vi "PCO_whisker_puff_pupil_FLIR_trig_2024_JMR.vi"() -> ()   [LabVIEW 2020]
uses:
  C:/Users/jqr5792/AppData/Roaming/PCO Digital Camera Toolbox/pco.labview/pco.camera/Controls/binning.ctl
  <vilib>/vision/driver/IMAQdx.llb/IMAQdx Camera Control Mode.ctl
  <vilib>/userDefined/High Color/IMAQdx.ctl
  <vilib>/vision/driver/IMAQdx.llb/IMAQdx Acquisition Mode.ctl
  C:/Users/jqr5792/AppData/Roaming/PCO Digital Camera Toolbox/pco.labview/pco.camera/Camera.lvclass
  <vilib>/vision/driver/IMAQdx.llb/IMAQdx Buffer Number Mode.ctl
  <vilib>/DAQmx/write.llb/DAQmx Write (Digital Bool 1Line 1Point).vi
  <vilib>/DAQmx/read.llb/DAQmx Read (Analog 1D Wfm NChan NSamp).vi
  <vilib>/DAQmx/write.llb/DAQmx Write (Digital 1D Bool NChan 1Samp 1Line).vi
  <vilib>/DAQmx/create/channels.llb/DAQmx Create Channel (AI-Voltage-Basic).vi
  <vilib>/DAQmx/configure/timing.llb/DAQmx Timing (Sample Clock).vi
  <vilib>/DAQmx/configure/trigger.llb/DAQmx Start Trigger (Digital Edge).vi
  <vilib>/DAQmx/create/channels.llb/DAQmx Create Channel (DO-Digital Output).vi
  <vilib>/DAQmx/create/channels.llb/DAQmx Create Channel (CO-Pulse Generation-Frequency).vi
  <vilib>/DAQmx/configure/timing.llb/DAQmx Timing (Implicit).vi
  <vilib>/DAQmx/miscellaneous.llb/DAQmx Fill In Error Info.vi
  <vilib>/vision/driver/NI_Vision_Acquisition_Software.lvlib
panel:
  out "n total images":i32
  out "PCO Frame Rate":dbl
  out "Time Elapsed (s)":u32
  out "Recorded Images":u32=7194
  out "PCO Recording":bool=TRUE
  in  "ROI":cluster{"x0":u64, "y0":u64, "x1":u64, "y1":u64}={"x0"=100, "y0"=175, "x1"=500, "y1"=425}
  in  "Binning":T1={"vert"=4, "horz"=4}
  in  "TriggerMode":T2(ring)=enum."external exposure start"
  in  "Exposure [s]":dbl=0.008 min=0.0005 max=2.0 step=0.001
  out "Image":T3(plugin-control)
  out "Last Whisk\nBuffer":u32=488
  out "Actual WhiskCam\nFrame Rate":dbl(knob)=148.05583250249254 scale=0.0..300.0
  out "Pupil":T3(plugin-control)
  out "Solenoids":bool[](array[boolean])
  in  "Stim \nOffset (s)":dbl=15.0
  in  "Stim \nDuration (s)":dbl=0.1 step=0.1
  in  "Inter-Stim\nInterval (s)":dbl=30.0
  in  "Right Pad 2":dbl=1.0
  in  "Left Pad 2":dbl=5.0
  in  "Control 2":dbl=2.0
  in  "Left Pad":tag="Dev1/port0/line1"
  in  "Right Pad":tag="Dev1/port0/line3"
  in  "Control":tag="Dev1/port0/line2"
  out "Analog Data":bool
  out "Analog acquisition length":i32
  in  "Channel Labels":string[](array[string])=["BallVelocity", "LeftPad", "Control", "RightPad", "Broadband", "LFP", "MUA"]
  in  "physical channels":tag="Dev1/ai0:6"
  in  "Analog Acquisition Setup":cluster{"Analog Sampling Rate":u16}={"Analog Sampling Rate"=5000} {"Analog Sampling Rate" format="%0.0f"}
  in  "Camera Acquisition Setup":cluster{"CBVCam Rate":u16, "WebCam Rate":u16}={"CBVCam Rate"=60, "WebCam Rate"=30}
  out "Notes Size":i32=7
  out "Notes Reversed":string[](array[string])=["Experimenter", "Animal ID", "Imaged Hemisphere", "Solenoid Pressure", "Isoflurane time", "Session ID", "Amplifier Gain"]
  out "Notes Array":string[](array[string])=["Amplifier Gain", "Session ID", "Isoflurane time", "Solenoid Pressure", "Imaged Hemisphere", "Animal ID", "Experimenter"]
  in  "Session Notes:":T4={"Experimenter"="Joe Ricotta", "Animal ID"="T31", "Imaged Hemisphere"="RH", "Solenoid Pressure"="10", "Infusion Compound"="na", "Infusion volume nL"="na", "Infusion rate nlpS"="na", "Block"="1000", "Molar conc um"="na"}
  in  "Target Path":path=path "D:/Joe/sample/PCO_setup" caption="Final saved file location"
  out "Current file name":string="170828_12_37_58"
  out "Actual WebCam Frame Rate":dbl(knob) scale=0.0..30.0
  out "WebCam":T3(plugin-control)
  out "CBV Camera":bool=TRUE
  out "Trial Time Elapsed (Min)":cluster{dbl, dbl}(slide)={0.5, 0.05364406000000001} scale=0.0..20.0
  in  "Recording Time (min)":dbl(knob)=5.0 min=0.5 max=25.0 step=0.5 scale=0.0..25.0 scale format="%#_2g"
  in  "Temp Path":path=path "C:/LabView Direct Files" caption="Temporary path for\nstreamed data"
  in  "Stop":bool
  # "File Settings:"
  # "Binning: 4,4"
  # "roi: 50, 200, 600, 400"
  # "Left Pad"
  # "Control"
  # "Right"
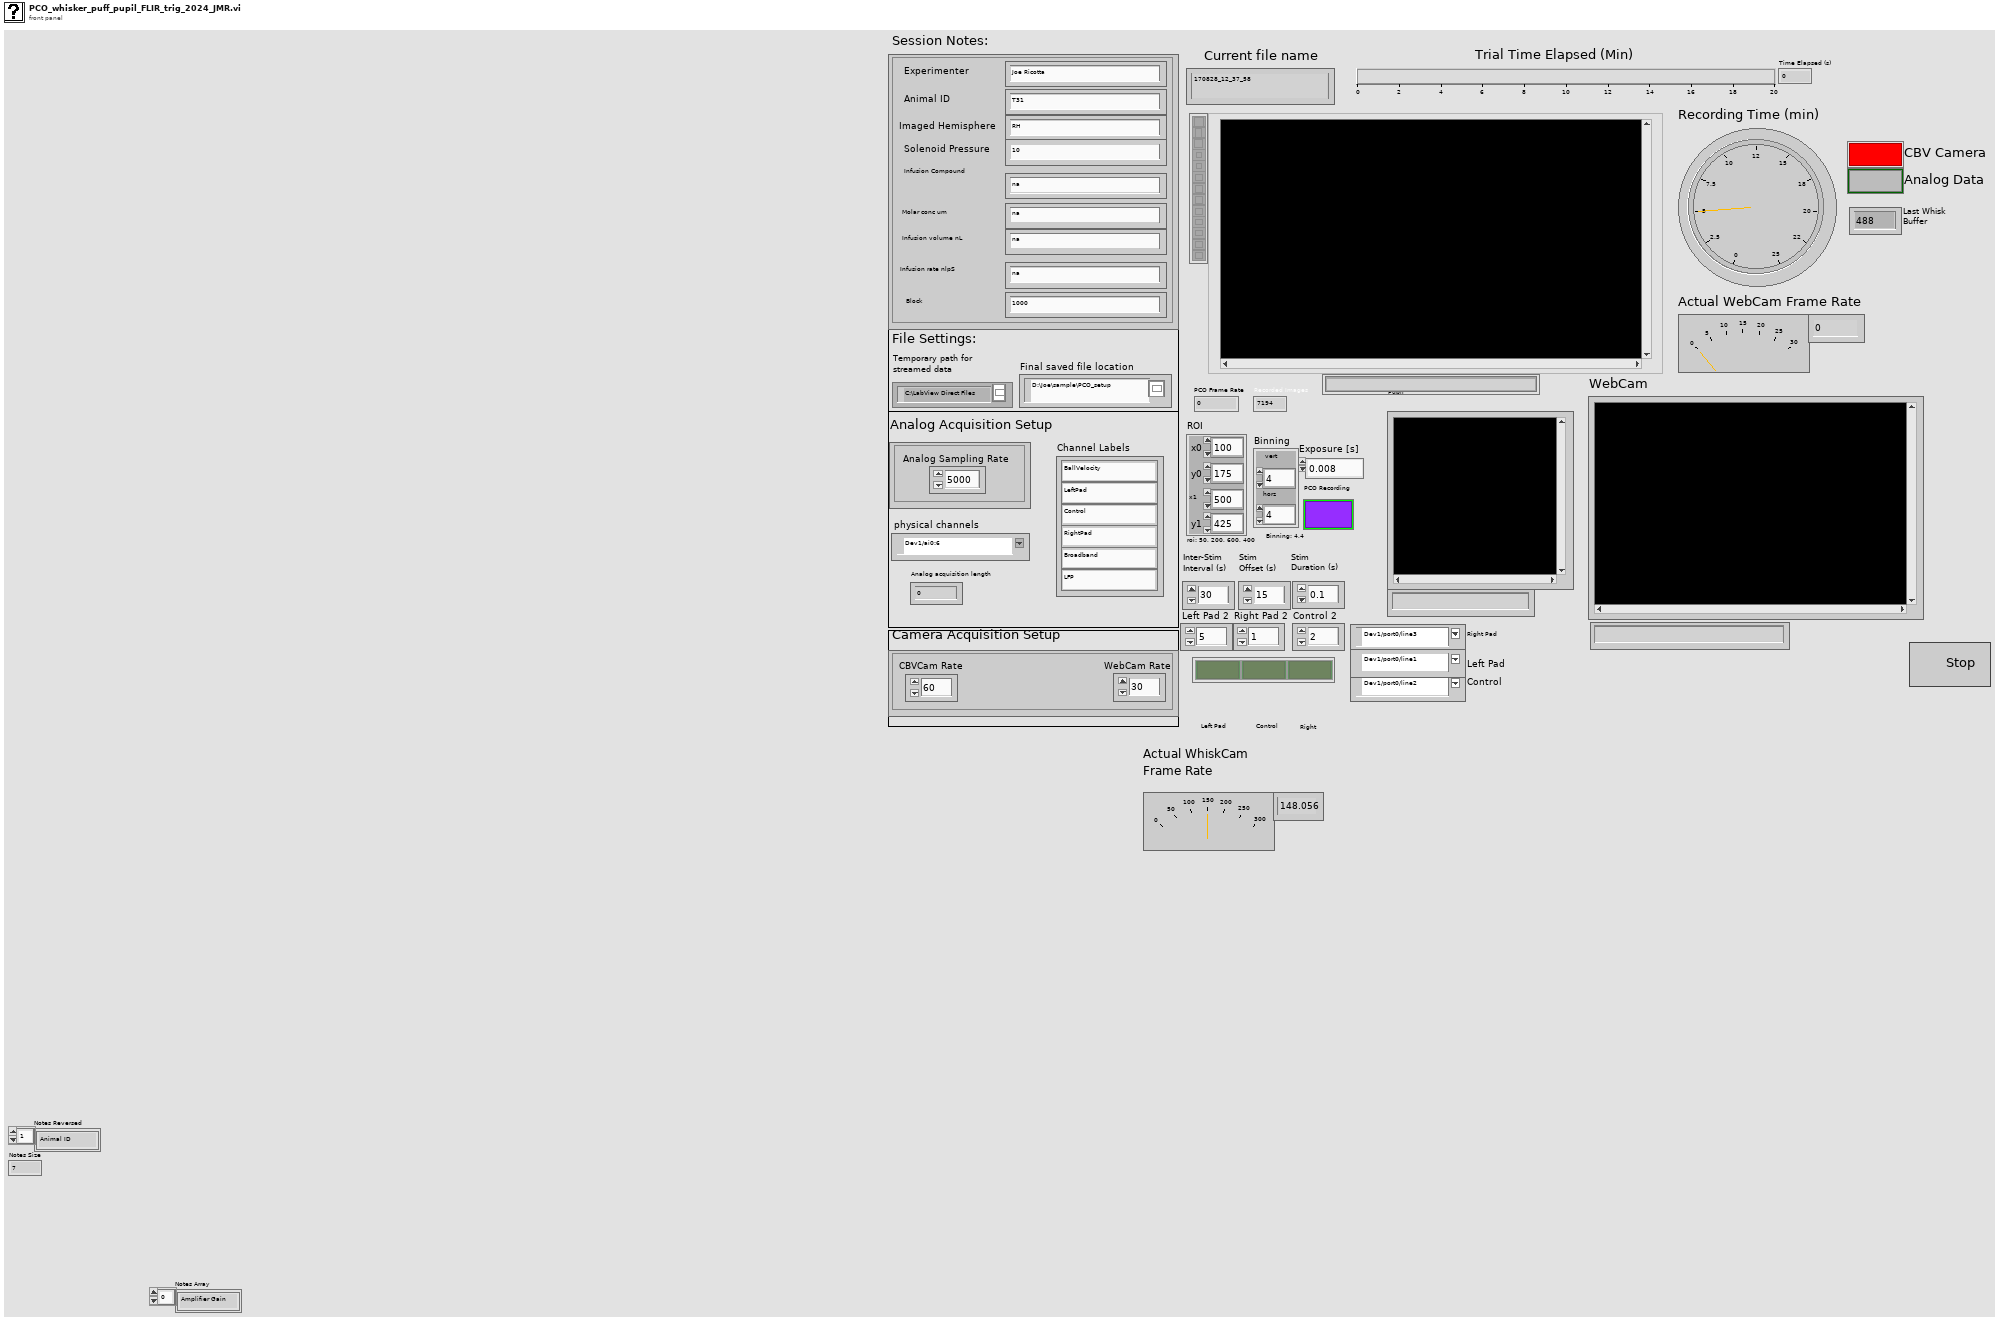
[diagram p1: front panel]
types:
  T1 = typedef "Camera.lvclass/binning.ctl" = cluster{"vert":u16, "horz":u16}
  T2 = enum16{"auto sequence", "software trigger", "external exposure start", "external exposure control"}
  T3 = typedef "IMAQ Image.ctl" = refnum<image>
  T4 = cluster{"Experimenter":string, "Animal ID":string, "Imaged Hemisphere":string, "Solenoid Pressure":string, "Infusion Compound":string, "Infusion volume nL":string, "Infusion rate nlpS":string, "Block":string, "Molar conc um":string}
  T5 = typedef "IMAQdx.ctl" = refnum<k21>
  T6 = typedef "Image Type" = u32
  T7 = enum16{"open", "replace", "create", "open or create", "replace or create", "replace or create with confirmation"}
  T8 = typedef "NI_Vision_Acquisition_Software.lvlib/IMAQdx Acquisition Mode.ctl" = enum32{"One Shot", "Continuous"}
  T9 = typedef "NI_Vision_Acquisition_Software.lvlib/IMAQdx Camera Control Mode.ctl" = enum32{"Controller", "Listener"}
  T10 = enum16{"open", "open or create", "create or replace", "create", "open (read-only)"}
  T11 = cluster{"exposure_time_s":dbl, "delay_time_s":dbl, "roi":cluster{"x0":u64, "y0":u64, "x1":u64, "y1":u64}, "timestamp_mode":u16, "pixelrate":u32, "trigger_mode":u16, "acquire_mode":u16, "metadata_mode":u16, "noisefilter_mode":u16, "binning":T1}
  T12 = typedef "IMAQ AVI2 Refnum.ctl" = refnum<k20>
  T13 = enum16{"sequence", "sequence non blocking", "ring buffer", "fifo", "sequence_dpcore", "sequence_non_blocking_dpcore", "ring_buffer_dpcore", "fifo_dpcore", "tif", "multitif", "pcoraw", "b16", "dicom", "multidicom"}
  T14 = enum16{"Undefined", "Mono8", "Mono16", "BGRA8", "RGBA8", "BGRA16", "RGBA16", "CompressedMono8"}
  T15 = enum16{"big-endian, network order", "native, host order", "little-endian"}
  T16 = typedef "NI_Vision_Acquisition_Software.lvlib/IMAQdx Buffer Number Mode.ctl" = enum32{"Next", "Last", "Buffer Number", "Every", "Last New"}
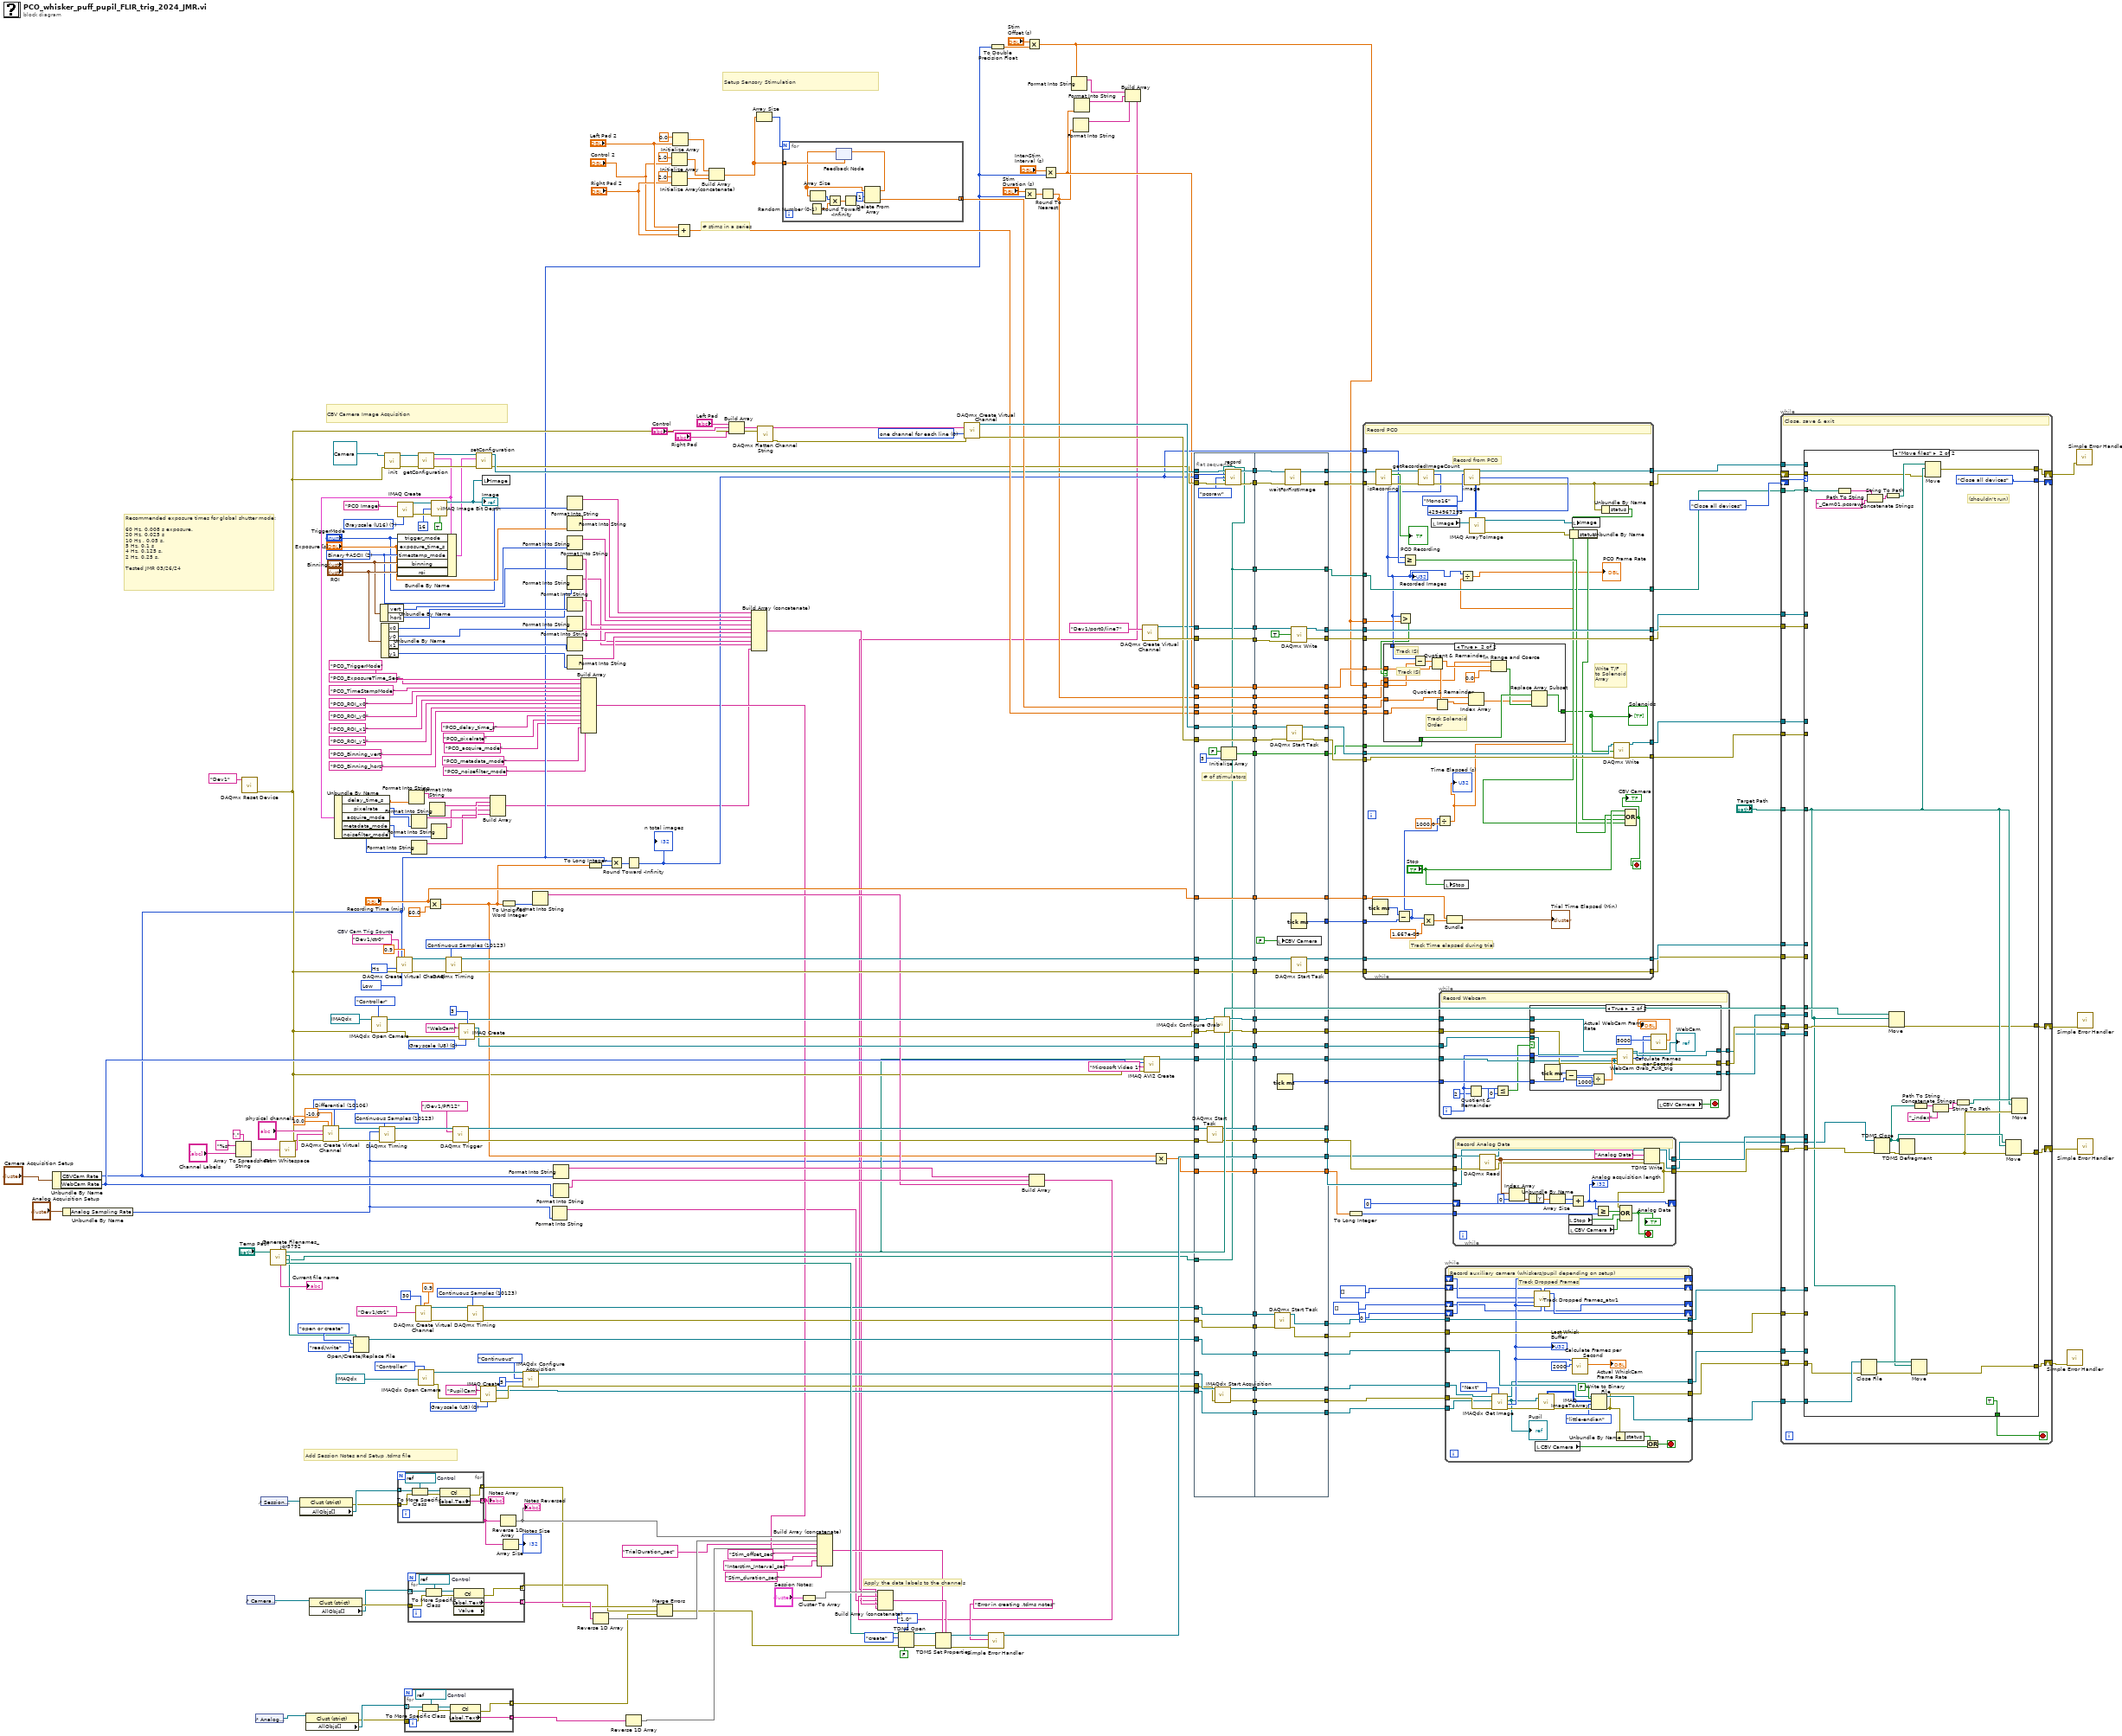
[diagram p0: block diagram]
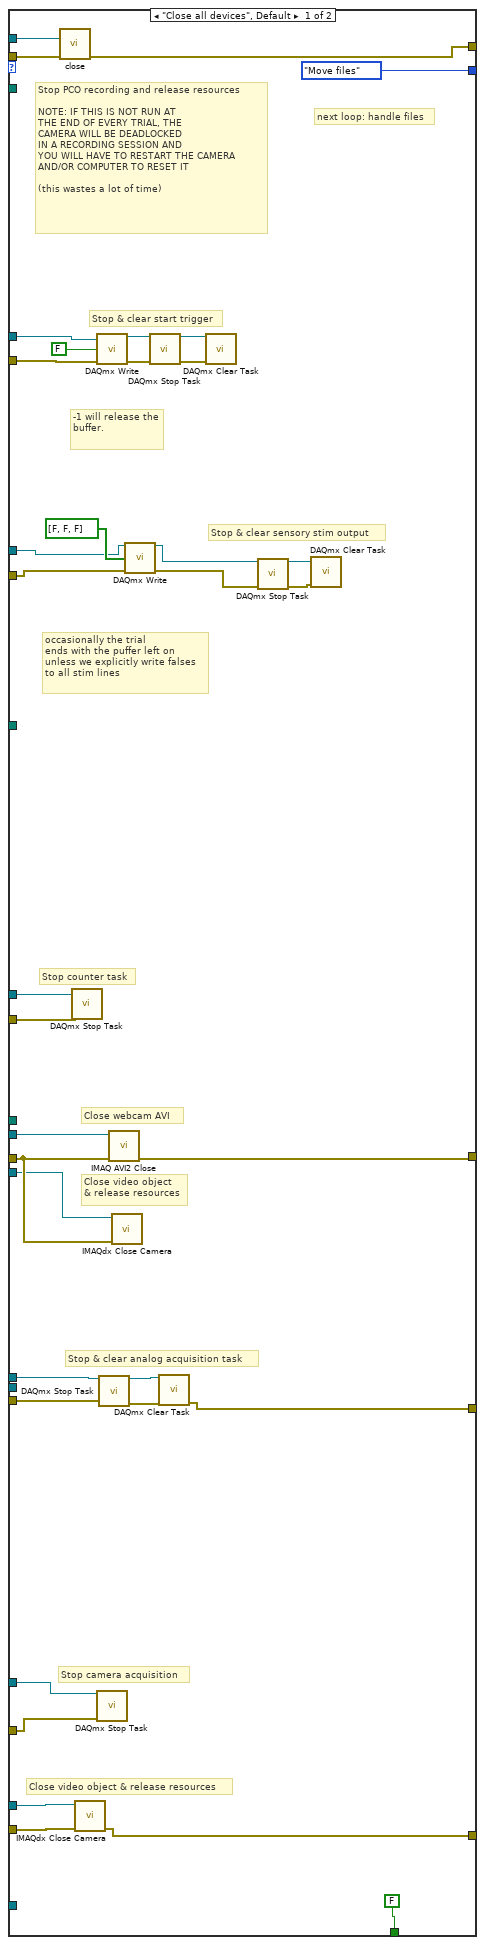
[diagram p2: hidden frame]
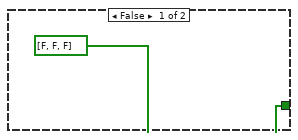
[diagram p4: hidden frame]
diagram:
  w84 = u16 2 items=["OFF", "Binary", "Binary+ASCII", "ASCII"] ("wTimeStampMode")
  w118 = T6 7 items=["Grayscale (U8)", "Grayscale (I16)", "Grayscale (SGL)", "Complex (CSG)", "RGB (U32)", "HSL (U32)", "RGB (U64)", "Grayscale (U16)"] ("Image Type")
  w148 = 10123 items=["Finite Samples"=10178, "Continuous Samples"=10123, "Hardware Timed Single Point"=12522] ("sample mode")
  w153 = T6 0 items=["Grayscale (U8)", "Grayscale (I16)", "Grayscale (SGL)", "Complex (CSG)", "RGB (U32)", "HSL (U32)", "RGB (U64)", "Grayscale (U16)"] ("Image Type")
  w203 = 0 items=["one channel for each line", "one channel for all lines"] ("line grouping")
  w206 = tag "Dev1/ctr0"  # CBV Cam Trig Source
  w280 = 10123 items=["Finite Samples"=10178, "Continuous Samples"=10123, "Hardware Timed Single Point"=12522] ("sample mode")
  w283 = 10106 items=["default"=-1, "RSE"=10083, "NRSE"=10078, "Differential"=10106, "Pseudodifferential"=12529] ("input terminal configuration")
  w303 = T6 0 items=["Grayscale (U8)", "Grayscale (I16)", "Grayscale (SGL)", "Complex (CSG)", "RGB (U32)", "HSL (U32)", "RGB (U64)", "Grayscale (U16)"] ("Image Type")
  w309 = 10123 items=["Finite Samples"=10178, "Continuous Samples"=10123, "Hardware Timed Single Point"=12522] ("sample mode")
  w312 = 10373 items=["Hz"=10373] ("units")
  w313 = 10214 items=["High"=10192, "Low"=10214] ("idle state")
  # "Recommended exposure times for global shutter mode:\n\n60 Hz, 0.008 s exposure.\n20 Hz, 0.025 s\n10 Hz , 0.05 s.\n5 Hz, 0.1 s\n4 Hz, 0.125 s.\n2 Hz, 0.25 s.\n\nTested JMR 03/26/24"
  # "Setup Sensory Stimulation"
  # "# stims in a series"
  # "Apply the data labels to the channels"
  # "CBV Camera Image Acquisition"
  # "Add Session Notes and Setup .tdms file"
  n1 = Unbundle By Name "Unbundle By Name"("Camera Acquisition Setup") -> ("CBVCam Rate"=w31:u16, "WebCam Rate"=w124:u16)
  n2 = Unbundle By Name("Analog Acquisition Setup") -> ("Analog Sampling Rate"=w29:u16)
  n3 = Array To Spreadsheet String(delimiter (Tab)=",", array="Channel Labels", 3:"%s" ("format string")) -> (spreadsheet string=w221:string)
  n4 = call <vilib>:"DAQmx Reset Device.vi"("device in"=tag "Dev1") -> ("error out"=w66:errorcluster)  [unwired: 14 in]
  n5 = control-ref of="Camera Acquisition Setup"() -> (w234:refnum<vi>)
  n6 = control-ref of="Analog Acquisition Setup"() -> (w233:refnum<vi>)
  n7 = control-ref of="Session Notes:"() -> (w257:refnum<vi>)
  n8 = call "Generate Filenames_jqr5792.vi"("path"="Temp Path") -> ("TDMS Path"=w251:path, "PCO Path"=w77:path, "Basler Path"=w145:path, "WebCam Path"=w44:path, "Analog file name"=→"Current file name":string)  [unwired: 5 in, 1 out]
  n9 = call <vilib>:"Trim Whitespace.vi"("string"=w221) -> ("trimmed string"=w220:string)  [unwired: 1 in]
  n10 = property class="Clust (strict)"(reference=w257) -> (error out=w260:errorcluster, "AllObjs[]"=w261:refnum<vi>[])  [unwired: 1 in, 1 out]
  n11 = property class="Clust (strict)"(reference=w233) -> (error out=w231:errorcluster, "AllObjs[]"=w232:refnum<vi>[])  [unwired: 1 in, 1 out]
  n12 = property class="Clust (strict)"(reference=w234) -> (error out=w255:errorcluster, "AllObjs[]"=w254:refnum<vi>[])  [unwired: 1 in, 1 out]
  n13 = call-poly <vilib>:"DAQmx Create Virtual Channel.vi"("maximum value"=10.0, "minimum value"=-10.0, "input terminal configuration"=w283, "physical channels"="physical channels", "name to assign"=w220, "error in"=w66) -> ("task out"=w282:refnum<k21>, "error out"=w281:errorcluster)  [unwired: 8 in]
  n14 = Open/Create/Replace File(file path (use dialog)=w145, operation (0:open)=T7."open or create", access (0:read/write)=enum16{"read/write", "read-only", "write-only"}."read/write") -> (refnum out=w129:refnum<file>)  [unwired: 3 in, 2 out]
  n15 = call <vilib>:"IMAQdx Open Camera.vi"("Camera Control Mode"=IMAQdx_Camera_Control_Mode."Controller", "error in"=w66, "Session In"=T5 "cam9") -> ("error out"=w300:errorcluster, "Session Out"=w298:T5)  [unwired: 7 in]
  n16 = call-poly <vilib>:"DAQmx Timing.vi"("task/channels in"=w282, "sample mode"=w280, "rate"=w29, "error in"=w281) -> ("task out"=w279:refnum<k21>, "error out"=w278:errorcluster)  [unwired: 10 in]
  n17 = Unbundle By Name("Binning") -> ("vert"=w85:u16, "horz"=w86:u16)
  n18 = Unbundle By Name("ROI") -> ("x0"=w87:u64, "y0"=w88:u64, "x1"=w89:u64, "y1"=w90:u64)
  n19 = call-dynamic "init.vi"("Camera in"=refnum<class "Camera.lvclass"> refnum ("PCOCamera in"), "error in (no error)"=w66) -> ("Camera out"=w112:refnum<class "Camera.lvclass">, "error out"=w111:errorcluster)  [unwired: 7 in]
  n20 = call-poly <vilib>:"DAQmx Create Virtual Channel.vi"("frequency"=w31, "duty cycle"=0.9, "counter"=w206, "units"=w312, "error in"=w66, "idle state"=w313) -> ("task out"=w311:refnum<k21>, "error out"=w310:errorcluster)  [unwired: 8 in]
  n21 = call "IMAQ Create"("Image Name"="PCO Image", "Image Type"=w118) -> ("New Image"=w117:T3, "error out"=w116:errorcluster)  [unwired: 3 in]
  n22 = for {
    tunnel: [w318] -> w259 mode=indexing
    tunnel: w261 -> [w317] mode=indexing
    tunnel: w260 -> [w316]
    tunnel: [w314] -> w240 mode=indexing
    w319 = refnum<vi> refnum  # Control
    n23 = To More Specific Class(target class=w319, reference=w317, error in=w316) -> (specific class reference=w320:refnum<vi>, error out=w315:errorcluster)
    n24 = property class="Ctl"(reference=w320, error in=w315) -> (error out=w314:errorcluster, "Label.Text"=w318:string)  [unwired: 1 out]
  }
  "Notes Array" <- w259
  n25 = for {
    tunnel: [w325] -> w229 mode=indexing
    tunnel: w232 -> [w324] mode=indexing
    tunnel: w231 -> [w323]
    tunnel: [w321] -> w230 mode=indexing
    w326 = refnum<vi> refnum  # Control
    n26 = To More Specific Class(target class=w326, reference=w324, error in=w323) -> (specific class reference=w327:refnum<vi>, error out=w322:errorcluster)
    n27 = property class="Ctl"(reference=w327, error in=w322) -> (error out=w321:errorcluster, "Label.Text"=w325:string)  [unwired: 1 out]
  }
  n28 = for {
    tunnel: [w332] -> w256 mode=indexing
    tunnel: w254 -> [w331] mode=indexing
    tunnel: w255 -> [w330]
    tunnel: [w328] -> w239 mode=indexing
    w333 = refnum<vi> refnum  # Control
    n29 = To More Specific Class(target class=w333, reference=w331, error in=w330) -> (specific class reference=w334:refnum<vi>, error out=w329:errorcluster)
    n30 = property class="Ctl" props=["Label", "Text", "Value"](reference=w334, error in=w329) -> (error out=w328:errorcluster, "Label.Text"=w332:string)  [unwired: 2 out]
  }
  n31 = call-poly <vilib>:"DAQmx Create Virtual Channel.vi"("frequency"=30, "duty cycle"=0.9, "counter"=tag "Dev1/ctr1" ("Whisker Cam\nTrigger Source")) -> ("task out"=w150:refnum<k21>, "error out"=w149:errorcluster)  [unwired: 11 in]
  n32 = call-dynamic "getConfiguration.vi"("error in (no error)"=w111, "Camera in"=w112) -> ("error out"=w110:errorcluster, "configuration"=w27:T11, "Camera out"=w113:refnum<class "Camera.lvclass">)  [unwired: 7 in]
  n33 = Unbundle By Name(w27) -> ("delay_time_s"=w21:dbl, "pixelrate"=w20:u32, "acquire_mode"=w19:u16, "metadata_mode"=w18:u16, "noisefilter_mode"=w17:u16)
  n34 = Bundle By Name(cluster=w27, "trigger_mode"="TriggerMode", "exposure_time_s"="Exposure [s]", "timestamp_mode"=w84, "binning"="Binning", "roi"="ROI") -> (w109:T11)
  n35 = Format Into String(w21) -> (resulting string=w16:string)  [unwired: 3 in, 1 out]
  n36 = Format Into String(w17) -> (resulting string=w12:string)  [unwired: 3 in, 1 out]
  n37 = Format Into String(w19) -> (resulting string=w14:string)  [unwired: 3 in, 1 out]
  n38 = call <vilib>:"IMAQdx Open Camera.vi"("Camera Control Mode"=IMAQdx_Camera_Control_Mode."Controller", "Session In"=T5 "cam5" ("Pupil Cam")) -> ("error out"=w156:errorcluster, "Session Out"=w159:T5)  [unwired: 8 in]
  n39 = Multiply(x="Recording Time (min)", y=60.0) -> (x*y=w72:dbl)
  n40 = Format Into String(w20) -> (resulting string=w15:string)  [unwired: 3 in, 1 out]
  n41 = call "IMAQ Image Bit Depth"("Image"=w117, "Bit Depth (0)"=u32 16, "error in (no error)"=w116, "Get/Set Bit Depth? (Set)"=TRUE) -> ("Image Out"=w119:T3)  [unwired: 9 in, 2 out]
  "Image" <- w119
  n42 = Format Into String(w18) -> (resulting string=w13:string)  [unwired: 3 in, 1 out]
  n43 = call-poly <vilib>:"DAQmx Timing.vi"("task/channels in"=w311, "sample mode"=w309, "error in"=w310) -> ("task out"=w267:refnum<k21>, "error out"=w265:errorcluster)  [unwired: 11 in]
  n44 = call-poly <vilib>:"DAQmx Trigger.vi"("task/channels in"=w279, "source"=tag "/Dev1/PFI12", "error in"=w278) -> ("task out"=w276:refnum<k21>, "error out"=w275:errorcluster)  [unwired: 11 in]
  n45 = call "IMAQ Create"("Border Size"=3, "Image Name"="WebCam", "Image Type"=w303, "error in (no error)"=w300) -> ("New Image"=w297:T3, "error out"=w299:errorcluster)  [unwired: 1 in]
  n46 = call-poly <vilib>:"DAQmx Timing.vi"("task/channels in"=w150, "sample mode"=w148, "error in"=w149) -> ("task out"=w138:refnum<k21>, "error out"=w136:errorcluster)  [unwired: 11 in]
  n47 = call-dynamic "setConfiguration.vi"("error in (no error)"=w110, "configuration"=w109, "Camera in"=w113) -> ("error out"=w78:errorcluster, "Camera out"=w79:refnum<class "Camera.lvclass">)  [unwired: 7 in]
  n48 = call "IMAQ Create"("Image Name"="PupilCam", "Image Type"=w153, "error in (no error)"=w156) -> ("New Image"=w132:T3, "error out"=w154:errorcluster)  [unwired: 2 in]
  n49 = local write "Image"(w119) -> ()
  n50 = Build Array(w16, w15, w14, w13, w12) -> (w11:string[])
  n51 = Reverse 1D Array(array=w259) -> (reversed array=w245:string[])
  "Notes Reversed" <- w245
  n52 = To Unsigned Word Integer(number=w72) -> (unsigned 16bit integer=w216:u16)
  n53 = Array Size(array=w259) -> (size(s)=→"Notes Size":i32)
  n54 = call <vilib>:"IMAQdx Configure Acquisition.vi"("error in"=w154, "Number of Buffers"=u32 5, "Continuous?"=IMAQdx_Acquisition_Mode."Continuous", "Session In"=w159) -> ("error out"=w133:errorcluster, "Session Out"=w134:T5)  [unwired: 6 in]
  n55 = Format Into String(w216) -> (resulting string=w217:string)  [unwired: 3 in, 1 out]
  n56 = Format Into String(w29) -> (resulting string=w28:string)  [unwired: 3 in, 1 out]
  n57 = Format Into String(w31) -> (resulting string=w227:string)  [unwired: 3 in, 1 out]
  n58 = Format Into String(w124) -> (resulting string=w226:string)  [unwired: 3 in, 1 out]
  n59 = Format Into String("TriggerMode") -> (resulting string=w97:string)  [unwired: 3 in, 1 out]
  n60 = Format Into String("Exposure [s]") -> (resulting string=w96:string)  [unwired: 3 in, 1 out]
  n61 = Format Into String(w84) -> (resulting string=w95:string)  [unwired: 3 in, 1 out]
  n62 = Format Into String(w85) -> (resulting string=w81:string)  [unwired: 3 in, 1 out]
  n63 = Format Into String(w86) -> (resulting string=w80:string)  [unwired: 3 in, 1 out]
  n64 = Format Into String(w87) -> (resulting string=w94:string)  [unwired: 3 in, 1 out]
  n65 = Format Into String(w88) -> (resulting string=w93:string)  [unwired: 3 in, 1 out]
  n66 = Format Into String(w89) -> (resulting string=w92:string)  [unwired: 3 in, 1 out]
  n67 = Format Into String(w90) -> (resulting string=w91:string)  [unwired: 3 in, 1 out]
  n68 = Build Array("PCO_TriggerMode", "PCO_ExposureTime_Sec", "PCO_TimeStampMode", "PCO_ROI_x0", "PCO_ROI_y0", "PCO_ROI_x1", "PCO_ROI_y1", "PCO_Binning_vert", "PCO_Binning_horz", "PCO_delay_time_s", "PCO_pixelrate", "PCO_acquire_mode", "PCO_metadata_mode", "PCO_noisefilter_mode") -> (w34:string[])
  n69 = To Long Integer(number=w72) -> (32bit integer=w71:i32)
  n70 = Reverse 1D Array(array=w256) -> (reversed array=w244:string[])
  n71 = Multiply(x=w31, y=w71) -> (x*y=w70:i32)
  n72 = Round Toward -Infinity(1:w70) -> (0:w69:i32)
  "n total images" <- w69
  n73 = Reverse 1D Array(array=w229) -> (reversed array=w228:string[])
  n74 = Merge Errors(w240, w239, w230) -> (w238:errorcluster)
  n75 = Initialize Array(1.0 ("element"), "Control 2") -> (w198:dbl[])
  n76 = Initialize Array(2.0 ("element"), "Right Pad 2") -> (w197:dbl[])
  n77 = Initialize Array(0.0 ("element"), "Left Pad 2") -> (w199:dbl[])
  n78 = Compound Arithmetic op=ADD("Left Pad 2", "Control 2", "Right Pad 2") -> (w173:dbl)
  n79 = Build Array (concatenate)(w199, w198, w197) -> (w196:dbl[])
  n80 = Build Array("Left Pad", "Control", "Right Pad") -> (w204:tag[])
  n81 = Build Array (concatenate)(w97, w96, w95, w94, w93, w92, w91, w81, w80, w11) -> (w33:string[])
  n82 = Array Size(array=w196) -> (size(s)=w190:i32)
  n83 = call <vilib>:"DAQmx Flatten Channel String.vi"("names in"=w204, "error in"=w66) -> ("names out"=w168:string, "error out"=w169:errorcluster)  [unwired: 12 in]
  n84 = for {
    N: w190 -> [_]
    tunnel: w196 -> [w338]
    tunnel: [w335] -> w176 mode=concatenating
    n85 = Random Number (0-1)() -> (number: 0 to 1=w342:dbl)
    n86 = feedback #1(w338) -> (w337:dbl[])
    n87 = Array Size(array=w337) -> (size(s)=w343:i32)
    n88 = Multiply(x=w343, y=w342) -> (x*y=w341:dbl)
    n89 = Round Toward -Infinity(1:w341) -> (0:w340:dbl)
    n90 = Delete From Array(array=w337, length=1, index=w340) -> (deleted portion=w335:dbl[], array with subset deleted=w336:dbl[])
    n91 = feedback-in #1(w336) -> ()
  }
  n92 = Cluster To Array(cluster="Session Notes:") -> (array=w252:string[])
  n93 = Build Array (concatenate)(w245, w244, "TrialDuration_sec", w228, w34, "Stim_offset_sec" ("array"), "Interstim_Interval_sec" ("array"), "Stim_duration_sec" ("array")) -> (w242:string[])
  n94 = TDMS Open(6:FALSE ("disable buffering? (T)"), 7:enum16{"1.0", "2.0"}."1.0" ("file format version (2.0)"), 8:w238, 10:T10."create" ("operation (0:open)"), 11:w251) -> (0:w246:errorcluster, 3:w247:refnum<k34>)  [unwired: 2 in]
  n95 = call-poly <vilib>:"DAQmx Create Virtual Channel.vi"("lines"=w168, "line grouping"=w203, "error in"=w169) -> ("task out"=w188:refnum<k21>, "error out"=w186:errorcluster)  [unwired: 11 in]
  n96 = To Double Precision Float(number=w31) -> (double precision float=w191:dbl)
  n97 = Multiply(x="Stim \nDuration (s)", y=w31) -> (x*y=w192:dbl)
  n98 = Multiply(x="Stim \nOffset (s)", y=w191) -> (x*y=w7:dbl)
  n99 = Build Array(w227, w226, w217) -> (w225:string[])
  n100 = Round To Nearest(number=w192) -> (nearest integer value=w5:dbl)
  n101 = Multiply(x="Inter-Stim\nInterval (s)", y=w31) -> (x*y=w6:dbl)
  n102 = Format Into String(w7) -> (resulting string=w4:string)  [unwired: 3 in, 1 out]
  n103 = Format Into String(w5) -> (resulting string=w2:string)  [unwired: 3 in, 1 out]
  n104 = Format Into String(w6) -> (resulting string=w3:string)  [unwired: 3 in, 1 out]
  n105 = Build Array(w4, w3, w2) -> (w1:string[])
  n106 = Build Array (concatenate)(w252, w225, w28, w33, w1) -> (w243:string[])
  n107 = TDMS Set Properties(5:w243, 7:w242, 8:w246, 11:w247) -> (0:w237:errorcluster, 3:w241:refnum<k34>)  [unwired: 2 in, 2 out]
  n108 = call <vilib>:"Simple Error Handler.vi"("error source (\" \")"="Error in creating .tdms notes" ("error source (\" \")"), "error in (no error)"=w237) -> ()  [unwired: 3 in, 5 out]
  n109 = call-poly <vilib>:"DAQmx Create Virtual Channel.vi"("lines"=tag "Dev1/port0/line7") -> ("task out"=w63:refnum<k21>, "error out"=w209:errorcluster)  [unwired: 13 in]
  n110 = call "IMAQ AVI2 Create"("error in (no error)"=w66, "Codec"="Microsoft Video 1", "Frames Per Second"=w124, "AVI Path"=w44) -> ("AVI Refnum"=w123:T12)  [unwired: 6 in, 1 out]
  n111 = Multiply(x=w72, y=w29) -> (x*y=w214:dbl)
  n112 = flat-sequence {
    tunnel: w299 -> [w384]
    tunnel: w298 -> [w383]
    tunnel: w297 -> [w382]
    tunnel: [w382] -> w296
    tunnel: [w381] -> w294
    tunnel: [w380] -> w292
    tunnel: w123 -> [w379]
    tunnel: [w379] -> w290
    tunnel: "Recording Time (min)" -> [w378]
    tunnel: [w378] -> w284
    tunnel: w276 -> [w377]
    tunnel: w275 -> [w376]
    tunnel: [w375] -> w274
    tunnel: [w374] -> w273
    tunnel: [w373] -> w268
    tunnel: w241 -> [w373]
    tunnel: w267 -> [w372]
    tunnel: [w372] -> w266
    tunnel: w265 -> [w371]
    tunnel: [w371] -> w264
    tunnel: w214 -> [w370]
    tunnel: [w370] -> w213
    tunnel: w209 -> [w369]
    tunnel: [w369] -> w208
    tunnel: w188 -> [w368]
    tunnel: [w368] -> w187
    tunnel: w186 -> [w367]
    tunnel: [w367] -> w185
    tunnel: [w364] -> w182
    tunnel: [w363] -> w179
    tunnel: w6 -> [w363]
    tunnel: w5 -> [w362]
    tunnel: [w362] -> w178
    tunnel: w176 -> [w361]
    tunnel: [w361] -> w175
    tunnel: w173 -> [w360]
    tunnel: [w360] -> w172
    tunnel: [w359] -> w142
    tunnel: [w358] -> w140
    tunnel: w138 -> [w357]
    tunnel: [w357] -> w137
    tunnel: w136 -> [w356]
    tunnel: [w356] -> w135
    tunnel: w134 -> [w355]
    tunnel: [w354] -> _
    tunnel: w133 -> [w354]
    tunnel: w132 -> [w353]
    tunnel: [w353] -> w131
    tunnel: w129 -> [w352]
    tunnel: [w352] -> w128
    tunnel: w79 -> [w351]
    tunnel: w78 -> [w350]
    tunnel: w77 -> [w345]
    tunnel: [w348] -> w76
    tunnel: [w347] -> w75
    tunnel: w69 -> [w346]
    tunnel: [w345] -> w68
    tunnel: w63 -> [w344]
    tunnel: [w344] -> w62
    tunnel: [w427] -> w301
    tunnel: w296 -> [w426]
    tunnel: [w426] -> w295
    tunnel: w294 -> [w425]
    tunnel: [w425] -> w293
    tunnel: w292 -> [w424]
    tunnel: [w424] -> w291
    tunnel: w290 -> [w423]
    tunnel: [w423] -> w289
    tunnel: [w417] -> w288
    tunnel: [w416] -> w287
    tunnel: [w422] -> w286
    tunnel: [w421] -> w285
    tunnel: w284 -> [w421]
    tunnel: [w420] -> w271
    tunnel: w274 -> [w420]
    tunnel: [w419] -> w272
    tunnel: w273 -> [w419]
    tunnel: [w418] -> w269
    tunnel: w268 -> [w418]
    tunnel: w266 -> [w415]
    tunnel: w264 -> [w414]
    tunnel: w213 -> [w413]
    tunnel: [w413] -> w212
    tunnel: w208 -> [w389]
    tunnel: w187 -> [w411]
    tunnel: w185 -> [w410]
    tunnel: [w409] -> w184
    tunnel: [w408] -> w183
    tunnel: w182 -> [w407]
    tunnel: [w407] -> w181
    tunnel: [w406] -> w180
    tunnel: w179 -> [w406]
    tunnel: w178 -> [w405]
    tunnel: [w405] -> w177
    tunnel: w175 -> [w404]
    tunnel: [w404] -> w174
    tunnel: w172 -> [w403]
    tunnel: [w403] -> w171
    tunnel: [w402] -> w144
    tunnel: [w401] -> w143
    tunnel: w142 -> [w400]
    tunnel: [w400] -> w141
    tunnel: w140 -> [w399]
    tunnel: [w399] -> w139
    tunnel: w137 -> [w398]
    tunnel: w135 -> [w397]
    tunnel: w131 -> [w396]
    tunnel: [w396] -> w130
    tunnel: w128 -> [w395]
    tunnel: [w395] -> w127
    tunnel: w76 -> [w394]
    tunnel: w75 -> [w393]
    tunnel: [w392] -> w74
    tunnel: [w391] -> w73
    tunnel: [w390] -> w67
    tunnel: w68 -> [w390]
    tunnel: [w388] -> w65
    tunnel: [w387] -> w64
    tunnel: w62 -> [w385]
    frame #0 {
      # "# of stimulators"
      n113 = call <vilib>:"DAQmx Start Task.vi"("task/channels in"=w377, "error in"=w376) -> ("task out"=w375:refnum<k21>, "error out"=w374:errorcluster)  [unwired: 12 in]
      n114 = call <vilib>:"IMAQdx Configure Grab.vi"("error in"=w384, "Session In"=w383) -> ("error out"=w380:errorcluster, "Session Out"=w381:T5)  [unwired: 8 in]
      n115 = call <vilib>:"IMAQdx Start Acquisition.vi"("error in"=w354, "Session In"=w355) -> ("error out"=w358:errorcluster, "Session Out"=w359:T5)  [unwired: 8 in]
      n116 = Initialize Array(FALSE, 3 ("dimension size")) -> (w364:bool[])
      n117 = call-dynamic "record.vi"("Camera in"=w351, "num_images"=w346, "record_mode"=T13."pcoraw", "file_path"=w345, "error in (no error)"=w350) -> ("Camera out"=w348:refnum<class "Camera.lvclass">, "error out"=w347:errorcluster)  [unwired: 9 in]
    }
    frame #1 {
      n118 = call <vilib>:"DAQmx Start Task.vi"("task/channels in"=w398, "error in"=w397) -> ("task out"=w402:refnum<k21>, "error out"=w401:errorcluster)  [unwired: 12 in]
      n119 = local write "CBV Camera"(FALSE ("Finished Acquiring")) -> ()
      n120 = Tick Count (ms)() -> (millisecond timer value=w427:u32)
      n121 = call-dynamic "waitForFirstImage.vi"("error in (no error)"=w393, "Camera in"=w394) -> ("error out"=w391:errorcluster, "Camera out"=w392:refnum<class "Camera.lvclass">)  [unwired: 8 in]
      n122 = call <vilib>:"DAQmx Start Task.vi"("task/channels in"=w411, "error in"=w410) -> ("task out"=w409:refnum<k21>, "error out"=w408:errorcluster)  [unwired: 12 in]
      n123 = Tick Count (ms)() -> (millisecond timer value=w422:u32)
      n124 = call-poly <vilib>:"DAQmx Write.vi"("task/channels in"=w385, "data"=TRUE, "error in"=w389) -> ("task out"=w388:refnum<k21>, "error out"=w387:errorcluster)  [unwired: 10 in, 1 out]
      n125 = call <vilib>:"DAQmx Start Task.vi"("task/channels in"=w415, "error in"=w414) -> ("task out"=w417:refnum<k21>, "error out"=w416:errorcluster)  [unwired: 12 in]
    }
  }
  n126 = To Long Integer(number=w212) -> (32bit integer=w211:i32)
  n127 = while {
    tunnel: [w476] -> w53
    tunnel: w288 -> [w476]
    tunnel: [w475] -> w52
    tunnel: w287 -> [w475]
    tunnel: w286 -> [w474]
    tunnel: w285 -> [w473]
    tunnel: w65 -> [w468]
    tunnel: [w468] -> w57
    tunnel: [w467] -> w56
    tunnel: w64 -> [w467]
    tunnel: [w466] -> w55
    tunnel: [w465] -> w54
    tunnel: w184 -> [w464]
    tunnel: w183 -> [w463]
    tunnel: w181 -> [w429]
    tunnel: w7 -> [w462]
    tunnel: w180 -> [w461]
    tunnel: w177 -> [w460]
    tunnel: w174 -> [w459]
    tunnel: w171 -> [w458]
    tunnel: w74 -> [w457]
    tunnel: w73 -> [w456]
    tunnel: [w443] -> w59
    tunnel: [w444] -> w60
    tunnel: w69 -> [w442]
    tunnel: w67 -> [w438]
    tunnel: [w438] -> w58
    tunnel: w7 -> [w431]
    stop <- w470 stop-if-true
    # "Record from PCO"
    # "Write T/F \nto Solenoid\nArray"
    # "Track ISI"
    # "Track Time elapsed during trial"
    # "Record PCO"
    n128 = Tick Count (ms)() -> (millisecond timer value=w477:u32)
    n129 = call-dynamic "isRecording.vi"("Camera in"=w457, "error in (no error)"=w456) -> ("Camera out"=w455:refnum<class "Camera.lvclass">, "recording"=→"PCO Recording":bool, "error out"=w454:errorcluster)  [unwired: 11 in]
    n130 = Subtract(x=w477, y=w474) -> (x-y=w434:u32)
    n131 = call-dynamic "getRecordedImageCount.vi"("Camera in"=w455, "error in (no error)"=w454) -> ("Camera out"=w446:refnum<class "Camera.lvclass">, "recorded_image_count"=w432:u32, "error out"=w445:errorcluster)  [unwired: 11 in]
    "Recorded Images" <- w432
    n132 = Greater?(x=w432, y=w431) -> (0:w430:bool)
    n133 = case shown="True" w430 {
      tunnel: w461 -> [_ w492]
      tunnel: w460 -> [_ w482]
      tunnel: w462 -> [_ w480]
      tunnel: w458 -> [_ w489]
      tunnel: w459 -> [_ w488]
      tunnel: w432 -> [_ w481]
      tunnel: w429 -> [_ w487]
      tunnel: [bool[] [FALSE, FALSE, FALSE] ("output array") w484] -> w428
      frame False {
      }
      frame True {
        # "Track Solenoid\nOrder"
        # "Track ISI"
        n134 = Subtract(x=w481, y=w480) -> (x-y=w479:dbl)
        n135 = Quotient & Remainder(x=w479, y=w492) -> (x-y*floor(x/y)=w493:dbl, floor(x/y)=w490:dbl)
        n136 = Quotient & Remainder(x=w490, y=w489) -> (x-y*floor(x/y)=w491:dbl)  [unwired: 1 out]
        n137 = Index Array(array=w488, index=w491) -> (element=w485:dbl)
        n138 = In Range and Coerce(upper limit=w482, x=w493, lower limit=0.0) -> (In Range?=w486:bool)  [unwired: 1 out]
        n139 = Replace Array Subset(array=w487, new element=w486, index=w485) -> (w484:bool[])
      }
    }
    "Solenoids" <- w428
    n140 = Greater Or Equal?(x=w432, y=w442) -> (x >= y?=w441:bool)
    n141 = Multiply(x=w434, y=1.667e-05) -> (x*y=w436:dbl)
    n142 = local read "Image"() -> (w447:T3)
    n143 = Divide(x=w434, y=1000.0) -> (x/y=w433:dbl)
    "Time Elapsed (s)" <- w433
    n144 = local write "Stop"("Stop") -> ()
    n145 = Bundle("Recording Time (min)"=w473, w436) -> (→"Trial Time Elapsed (Min)":cluster{"Recording Time (min)":dbl, dbl})  [unwired: 1 in]
    n146 = Divide(x=w432, y=w433) -> (x/y=→"PCO Frame Rate":dbl)
    n147 = call-dynamic "image.vi"("Camera in"=w446, "data_format"=T14."Mono16", "image_index"=u32 4294967295 ("dwImgIdx"), "error in (no error)"=w445) -> ("Camera out"=w443:refnum<class "Camera.lvclass">, "raw_image (U16)"=w448:u16[][], "error out"=w444:errorcluster)  [unwired: 4 in, 5 out]
    n148 = call "IMAQ ArrayToImage"("Image Pixels (U16)"=w448, "Image"=w447) -> ("error out"=w450:errorcluster, "Image Out"=w452:T3)  [unwired: 8 in]
    n149 = Unbundle By Name(w450) -> ("status"=w440:bool)
    n150 = local write "Image"(w452) -> ()
    n151 = Unbundle By Name(w444) -> ("status"=w439:bool)
    n152 = call-poly <vilib>:"DAQmx Write.vi"("task/channels in"=w464, "data"=w428, "error in"=w463) -> ("task out"=w466:refnum<k21>, "error out"=w465:errorcluster)  [unwired: 10 in, 1 out]
    n153 = Compound Arithmetic op=OR("Stop", w441, w440, w439) -> (w470:bool)
    "CBV Camera" <- w470
  }
  n154 = while {
    tunnel: w301 -> [w506]
    tunnel: w295 -> [w499]
    tunnel: w293 -> [w505]
    tunnel: w291 -> [w504]
    tunnel: w289 -> [w500]
    tunnel: [w503] -> w49
    tunnel: [w502] -> w51
    tunnel: [w501] -> w50
    i -> [w498]
    stop <- w507 stop-if-true
    # "Record Webcam"
    n155 = Quotient & Remainder(x=w498, y=2) -> (x-y*floor(x/y)=w496:i32)  [unwired: 1 out]
    n156 = Less Or Equal?(x=w496, y=0) -> (x <= y?=w494:bool)
    n157 = case shown="True" w494 {
      tunnel: w506 -> [_ w521]
      tunnel: w505 -> [w510 w520]
      tunnel: w504 -> [w509 w516]
      tunnel: [w510 w515] -> w503
      tunnel: [w509 w513] -> w502
      tunnel: [w508 w511] -> w501
      tunnel: w500 -> [w508 w511]
      tunnel: w499 -> [_ w519]
      tunnel: w498 -> [_ w518]
      frame False {
      }
      frame True {
        n158 = Tick Count (ms)() -> (millisecond timer value=w524:u32)
        n159 = Subtract(x=w524, y=w521) -> (x-y=w525:u32)
        n160 = Divide(x=w525, y=u32 1000) -> (x/y=w517:dbl)
        n161 = call "WebCam Grab_FLIR_trig.vi"("Session In"=w520, "Image In"=w519, "Buffer Number In"=w518, "Trial Time"=w517, "AVI Refnum"=w511, "error in"=w516) -> ("Session Out"=w515:T5, "WebCam Img Out"=→"WebCam":T3, "Buffer Number Out"=w512:u32, "error out"=w513:errorcluster)  [unwired: 10 in]
        n162 = call <vilib>:"Calculate Frames per Second.vi"("Update Interval (ms)"=u32 5000, "Buffer Number"=w512) -> ("Processed Frames/s"=→"Actual WebCam Frame Rate":dbl)  [unwired: 7 in, 2 out]
      }
    }
    n163 = local read "CBV Camera"() -> (w507:bool)
  }
  n164 = while {
    tunnel: w144 -> [w546]
    tunnel: [w547] -> w45
    tunnel: w143 -> [w547]
    tunnel: [w546] -> w46
    tunnel: [w529] -> w47
    tunnel: [w531] -> w40
    tunnel: [w545] -> w39
    tunnel: w141 -> [w544]
    tunnel: w139 -> [w543]
    tunnel: w130 -> [w542]
    tunnel: w127 -> [w541]
    shift-right: [w540] -> _
    shift-left: _ -> [w539]
    shift-right: [w538] -> _
    shift-left: u32 0 ("New Lost") -> [w537]
    shift-right: [w536] -> _
    shift-left: u32[] [] ("NewBuffNum") -> [w535]
    shift-right: [w534] -> _
    shift-left: u32[] [] ("NewNumLost") -> [w533]
    stop <- w532 stop-if-true
    # "Track Dropped Frames"
    # "Record auxiliary camera (whiskers/pupil depending on setup)"
    n165 = call <vilib>:"IMAQdx Get Image.vi"("Buffer Number Mode (Next)"=IMAQdx_Buffer_Number_Mode."Next", "error in"=w543, "Image In"=w542, "Session In"=w544) -> ("error out"=w554:errorcluster, "Buffer Number Out"=w540:u32, "Image Out"=w527:T3, "Session Out"=w529:T5)  [unwired: 4 in]
    "Last Whisk\nBuffer" <- w540
    "Pupil" <- w527
    n166 = call "Track Dropped Frames_atw1.vi"("NumLost"=w533, "BuffNum"=w535, "Curr Buffer"=w540, "Prev Lost"=w537, "Prev Buffer"=w539) -> ("New Lost"=w538:u32, "NewNumLost"=w534:u32[], "NewBuffNum"=w536:u32[])  [unwired: 4 in]
    n167 = local read "CBV Camera"() -> (w528:bool)
    n168 = call "IMAQ ImageToArray"("error in (no error)"=w554, "Image"=w527) -> ("error out"=w553:errorcluster, "Image Pixels (U8)"=w552:u8[][])  [unwired: 2 in, 3 out]
    n169 = call <vilib>:"Calculate Frames per Second.vi"("Update Interval (ms)"=u32 2000, "Buffer Number"=w540) -> ("Processed Frames/s"=→"Actual WhiskCam\nFrame Rate":dbl)  [unwired: 7 in, 2 out]
    n170 = Write to Binary File(file (use dialog)=w541, data=w552, error in=w553, 5:FALSE ("prepend array or string size? (T)"), 9:T15."little-endian" ("byte order (0:big-endian, network order)")) -> (refnum out=w545:refnum<file>, error out=w531:errorcluster)  [unwired: 1 in, 1 out]
    n171 = Unbundle By Name(w531) -> ("status"=w530:bool)
    n172 = Or(x=w530, y=w528) -> (x .or. y?=w532:bool)
  }
  n173 = while {
    tunnel: w272 -> [w575]
    tunnel: w271 -> [w574]
    tunnel: w269 -> [w573]
    tunnel: [w572] -> w41
    tunnel: [w556] -> w42
    tunnel: [w571] -> w48
    shift-right: [w563] -> _
    shift-left: 0 -> [w564]
    tunnel: w211 -> [w562]
    stop <- w558 stop-if-true
    # "Record Analog Data"
    n174 = call-poly <vilib>:"DAQmx Read.vi"("task/channels in"=w574, "error in"=w575) -> ("task out"=w571:refnum<k21>, "data"=w569:waveform(dbl)[], "error out"=w561:errorcluster)  [unwired: 11 in]
    n175 = Index Array(array=w569, index=0) -> (element=w567:waveform(dbl))
    n176 = Unbundle By Name(w567) -> ("Y"=w566:dbl[])
    n177 = Array Size(array=w566) -> (size(s)=w565:i32)
    n178 = local read "Stop"() -> (w559:bool)
    n179 = local read "CBV Camera"() -> (w557:bool)
    n180 = Add(x=w565, y=w564) -> (x+y=w563:i32)
    "Analog acquisition length" <- w563
    n181 = Greater Or Equal?(x=w563, y=w562) -> (x >= y?=w560:bool)
    n182 = TDMS Write(0:w573, 5:"Analog Data" ("group name in (Untitled)"), 9:w569, 11:w561) -> (4:w572:refnum<k34>, 15:w556:errorcluster)  [unwired: 2 in, 2 out]
    n183 = Compound Arithmetic op=OR(w556, w560, w559, w557) -> (w558:bool)
    "Analog Data" <- w558
  }
  n184 = while {
    shift-right: [w603] -> _
    shift-left: enum16{"Close all devices", "Move files"}."Close all devices" ("Enum") -> [w604]
    tunnel: w59 -> [w601]
    tunnel: w58 -> [w600]
    tunnel: w57 -> [w599]
    tunnel: w56 -> [w598]
    tunnel: w55 -> [w597]
    tunnel: w54 -> [w596]
    tunnel: w53 -> [w595]
    tunnel: w52 -> [w594]
    tunnel: w50 -> [w592]
    tunnel: w49 -> [w591]
    tunnel: w48 -> [w590]
    tunnel: w47 -> [w587]
    tunnel: w46 -> [w586]
    tunnel: w45 -> [w585]
    tunnel: w44 -> [w584]
    shift-right: [w577] -> w36
    shift-left: w51 -> [w593]
    tunnel: "Target Path" -> [w583]
    tunnel: w41 -> [w582]
    shift-right: [w578] -> w37
    shift-left: w42 -> [w589]
    tunnel: w39 -> [w581]
    shift-right: [w579] -> w38
    shift-left: w40 -> [w588]
    shift-right: [w576] -> w35
    shift-left: w60 -> [w602]
    stop <- w580 stop-if-true
    # "Close, save & exit"
    n185 = case shown="\"Move files\"" w604 {
      tunnel: [enum16{"Close all devices", "Move files"}."Move files" ("Enum") enum16{"Close all devices", "Move files"}."Close all devices" ("Enum")] -> w603
      tunnel: w602 -> [w638 w641]
      tunnel: w601 -> [w637 _]
      tunnel: w600 -> [_ w663]
      tunnel: w599 -> [w632 _]
      tunnel: w598 -> [w630 _]
      tunnel: w597 -> [w608 _]
      tunnel: w596 -> [w606 _]
      tunnel: w595 -> [w627 _]
      tunnel: w594 -> [w626 _]
      tunnel: w593 -> [w624 w661]
      tunnel: w592 -> [w625 _]
      tunnel: w591 -> [w623 _]
      tunnel: w590 -> [w622 _]
      tunnel: w589 -> [w621 w653]
      tunnel: w588 -> [w619 w648]
      tunnel: w587 -> [w618 _]
      tunnel: w586 -> [w617 _]
      tunnel: w585 -> [w616 _]
      tunnel: w584 -> [_ w662]
      tunnel: w583 -> [_ w649]
      tunnel: w582 -> [_ w640]
      tunnel: w581 -> [_ w650]
      tunnel: [FALSE TRUE] -> w580
      tunnel: [w611 w645] -> w579
      tunnel: [w612 w644] -> w578
      tunnel: [w613 w643] -> w577
      tunnel: [w610 w642] -> w576
      frame "Close all devices", Default {
        # "occasionally the trial\nends with the puffer left on\nunless we explicitly write falses\nto all stim lines"
        # "next loop: handle files"
        # "Stop PCO recording and release resources\n\nNOTE: IF THIS IS NOT RUN AT \nTHE END OF EVERY TRIAL, THE\nCAMERA WILL BE DEADLOCKED\nIN A RECORDING SESSION AND \nYOU WILL HAVE TO RESTART THE CAMERA\nAND/OR COMPUTER TO RESET IT\n\n(this wastes a lot of time)"
        # "Stop & clear start trigger"
        # "Stop & clear sensory stim output"
        # "Stop counter task"
        # "Close video object\n& release resources"
        # "Close webcam AVI"
        # "Close video object & release resources"
        # "Stop camera acquisition"
        # "Stop & clear analog acquisition task"
        # "-1 will release the buffer."
        n186 = call-dynamic "close.vi"("error in (no error)"=w638, "Camera in"=w637) -> ("error out"=w610:errorcluster)  [unwired: 9 in]
        n187 = call <vilib>:"DAQmx Stop Task.vi"("task/channels in"=w627, "error in"=w626) -> ()  [unwired: 12 in, 2 out]
        n188 = call <vilib>:"IMAQdx Close Camera.vi"("error in"=w619, "Session In"=w618) -> ("error out"=w611:errorcluster)  [unwired: 9 in]
        n189 = call-poly <vilib>:"DAQmx Write.vi"("task/channels in"=w632, "data"=FALSE, "error in"=w630) -> ("task out"=w633:refnum<k21>, "error out"=w635:errorcluster)  [unwired: 10 in, 1 out]
        n190 = call <vilib>:"DAQmx Stop Task.vi"("task/channels in"=w617, "error in"=w616) -> ()  [unwired: 12 in, 2 out]
        n191 = call <vilib>:"DAQmx Stop Task.vi"("task/channels in"=w622, "error in"=w621) -> ("task out"=w620:refnum<k21>, "error out"=w615:errorcluster)  [unwired: 12 in]
        n192 = call "IMAQ AVI2 Close"("error in (no error)"=w624, "AVI Refnum"=w625) -> ("error out"=w613:errorcluster)  [unwired: 9 in]
        n193 = call <vilib>:"IMAQdx Close Camera.vi"("error in"=w624, "Session In"=w623) -> ()  [unwired: 9 in, 1 out]
        n194 = call-poly <vilib>:"DAQmx Write.vi"("task/channels in"=w608, "data"=bool[] [FALSE, FALSE, FALSE], "error in"=w606) -> ("task out"=w607:refnum<k21>, "error out"=w605:errorcluster)  [unwired: 10 in, 1 out]
        n195 = call <vilib>:"DAQmx Stop Task.vi"("task/channels in"=w633, "error in"=w635) -> ("task out"=w634:refnum<k21>, "error out"=w636:errorcluster)  [unwired: 12 in]
        n196 = call <vilib>:"DAQmx Clear Task.vi"("task in"=w620, "error in"=w615) -> ("error out"=w612:errorcluster)  [unwired: 13 in]
        n197 = call <vilib>:"DAQmx Clear Task.vi"("task in"=w634, "error in"=w636) -> ()  [unwired: 13 in, 1 out]
        n198 = call <vilib>:"DAQmx Stop Task.vi"("task/channels in"=w607, "error in"=w605) -> ("task out"=w629:refnum<k21>, "error out"=w628:errorcluster)  [unwired: 12 in]
        n199 = call <vilib>:"DAQmx Clear Task.vi"("task in"=w629, "error in"=w628) -> ()  [unwired: 13 in, 1 out]
      }
      frame "Move files" {
        # "(shouldn't run)"
        n200 = Path To String(path=w663) -> (string=w665:string)
        n201 = Close File(refnum=w650, error in=w648) -> (path=w651:path, error out=w652:errorcluster)
        n202 = Concatenate Strings(w665, "_Cam01.pcoraw" ("string")) -> (w666:string)
        n203 = TDMS Close(8:w653, 11:w640) -> (0:w655:errorcluster, 3:w657:path)
        n204 = String To Path(string=w666) -> (path=w667:path)
        n205 = Move(source path=w662, error in=w661, 10:w649) -> (error out=w643:errorcluster)  [unwired: 2 in, 2 out]
        n206 = TDMS Defragment(4:w655, 7:w657) -> (0:w660:errorcluster)
        n207 = Move(source path=w651, error in=w652, 10:w649) -> (error out=w645:errorcluster)  [unwired: 2 in, 2 out]
        n208 = Path To String(path=w657) -> (string=w656:string)
        n209 = Move(source path=w667, error in=w641, 10:w649) -> (error out=w642:errorcluster)  [unwired: 2 in, 2 out]
        n210 = Concatenate Strings(w656, "_index" ("string")) -> (w658:string)
        n211 = String To Path(string=w658) -> (path=w659:path)
        n212 = Move(source path=w657, error in=w660, 10:w649) -> (error out=w644:errorcluster)  [unwired: 2 in, 2 out]
        n213 = Move(source path=w659, error in=w660, 10:w649) -> ()  [unwired: 2 in, 3 out]
      }
    }
  }
  n214 = call <vilib>:"Simple Error Handler.vi"("error in (no error)"=w38) -> ()  [unwired: 1 in, 8 out]
  n215 = call <vilib>:"Simple Error Handler.vi"("error in (no error)"=w35) -> ()  [unwired: 1 in, 8 out]
  n216 = call <vilib>:"Simple Error Handler.vi"("error in (no error)"=w36) -> ()  [unwired: 1 in, 8 out]
  n217 = call <vilib>:"Simple Error Handler.vi"("error in (no error)"=w37) -> ()  [unwired: 1 in, 8 out]
